vi "ActionVIOnCompile.vi"(8 "error in (no error)":errorcluster, 11 "Device Item Ref in":T1 format="%.0x") -> (0 "error out":errorcluster)   [LabVIEW 2011, in "Chassis TimeSync System Explorer.lvlib"]
uses:
  Chassis TimeSync System Explorer.lvlib
  <vilib>/NI Veristand/Custom Device API/Custom Device Item Ref.ctl
  Shared/Compiled Data.ctl
  Shared/Connection Settings.ctl
  Shared/Mode.ctl
  Shared/External Pin.ctl
  Shared/Routes.ctl
  Shared/Route.ctl
  Shared/Time Ref Settings.ctl
  Shared/Time Reference.ctl
  Shared/IRIG Type.ctl
  Shared/Constants.vi
  <vilib>/NI Veristand/Custom Device API/Get Item Property (String).vi
  <vilib>/NI Veristand/Custom Device API/Get Item Property (U16).vi
  <vilib>/NI Veristand/Custom Device API/Get Item Property (Double).vi
  <vilib>/NI Veristand/Custom Device API/Get Item Property (Boolean).vi
  <vilib>/NI Veristand/Custom Device API/Set Item Property (Variant).vi
  Shared/Chassis TimeSync Shared.lvlib
  <vilib>/NI Veristand/Custom Device API/Custom Device API.lvlib
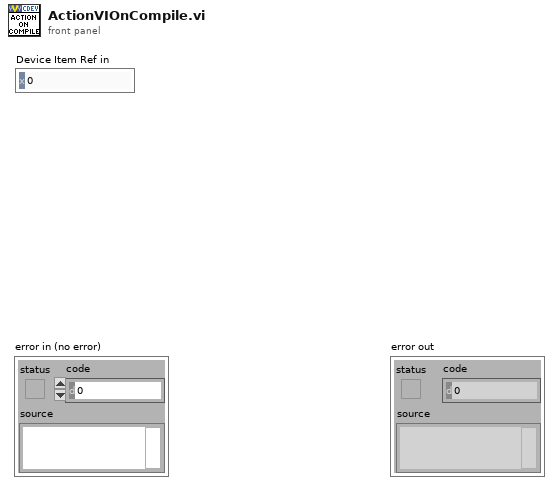
[diagram p1: front panel]
types:
  T1 = typedef "Custom Device API.lvlib/Custom Device Item Ref.ctl" = u64
  T2 = typedef "Chassis TimeSync Shared.lvlib/Compiled Data.ctl" = cluster{"SyncMod?":bool, "SyncMod":string, "ConnectionSettings":T3, "TimeKeeper":string, "ScanOffset(%)":dbl, "StartDelay(s)":u16, "Time Ref Settings":T8, "FIFO Locations":cluster{"SysTime":i32[], "TimeRef":i32[], "Status":i32[]}}
  T3 = typedef "Chassis TimeSync Shared.lvlib/Connection Settings.ctl" = cluster{"Mode":T4, "pxitrig":bool, "pfi0":bool, "pfi1":bool, "pfi2":bool, "External Pin":T5, "Routes":T6}
  T4 = typedef "Chassis TimeSync Shared.lvlib/Mode.ctl" = enum16{"Generate sample clock", "Route sample clock out of chassis", "Route sample clock into chassis", "Custom routes"}
  T5 = typedef "Chassis TimeSync Shared.lvlib/External Pin.ctl" = enum16{"PFI0", "PFI1", "PFI2"}
  T6 = typedef "Chassis TimeSync Shared.lvlib/Routes.ctl" = T7[]
  T7 = typedef "Chassis TimeSync Shared.lvlib/Route.ctl" = cluster{"Source":string, "Destination":string}
  T8 = typedef "Chassis TimeSync Shared.lvlib/Time Ref Settings.ctl" = cluster{"Time Reference":T9, "Priority 1":i32, "Priority 2":i32, "IRIG type":T10, "Terminal":string, "PPSSetTime":bool, "Start Time":timestamp}
  T9 = typedef "Chassis TimeSync Shared.lvlib/Time Reference.ctl" = enum16{"GPS", "IRIG", "PPS", "1588 Ordinary Clock", "PXI Chassis Clock"}
  T10 = typedef "Chassis TimeSync Shared.lvlib/IRIG Type.ctl" = enum16{"IRIGB DC", "IRIGB AM"}
  T11 = typedef "Chassis TimeSync Shared.lvlib/Channel.ctl" = cluster{"Name":string, "Units":string, "Default":dbl, "Description":string}
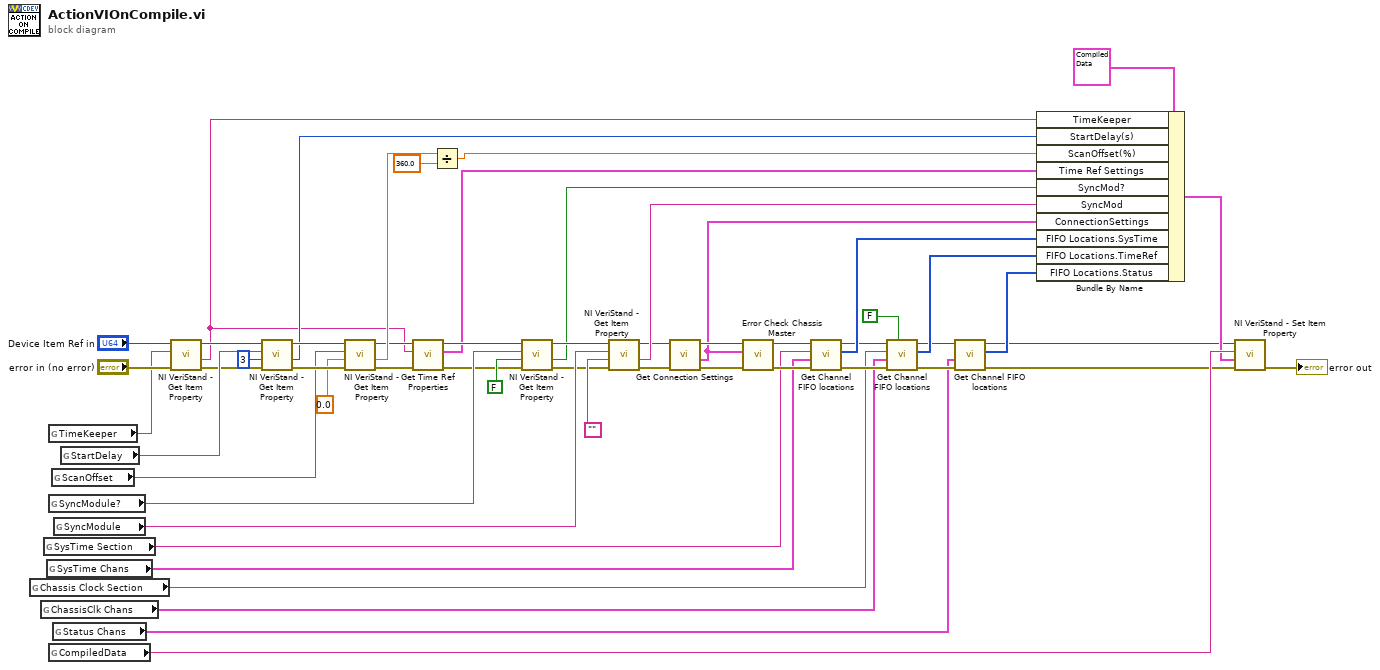
[diagram p0: block diagram]
diagram:
  n1 = global read "Constants.vi" "Chassis Clock Section"() -> (w11:string)
  n2 = global read "Constants.vi" "ChassisClk Chans"() -> (w10:T11[])
  n3 = global read "Constants.vi" "SysTime Section"() -> (w15:string)
  n4 = global read "Constants.vi" "SysTime Chans"() -> (w16:T11[])
  n5 = global read "Constants.vi" "TimeKeeper"() -> (w53:string)
  n6 = global read "Constants.vi" "SyncModule?"() -> (w37:string)
  n7 = global read "Constants.vi" "CompiledData"() -> (w20:string)
  n8 = global read "Constants.vi" "ScanOffset"() -> (w48:string)
  n9 = global read "Constants.vi" "Status Chans"() -> (w6:T11[])
  n10 = global read "Constants.vi" "SyncModule"() -> (w35:string)
  n11 = global read "Constants.vi" "StartDelay"() -> (w50:string)
  n12 = call-poly <vilib>:"NI VeriStand - Get Item Property.vi"("error in (no error)"="error in (no error)", "Property Name"=w53, "Item Ref in"="Device Item Ref in") -> ("error out"=w46:errorcluster, "Value"=w38:string, "Item Ref out"=w45:T1)  [unwired: 5 in, 1 out]
  n13 = call-poly <vilib>:"NI VeriStand - Get Item Property.vi"("error in (no error)"=w46, "Default Value"=u16 3 ("Start Offset Multiple"), "Property Name"=w50, "Item Ref in"=w45) -> ("error out"=w51:errorcluster, "Value"=w44:u16, "Item Ref out"=w52:T1)  [unwired: 4 in, 1 out]
  n14 = call-poly <vilib>:"NI VeriStand - Get Item Property.vi"("error in (no error)"=w51, "Default Value"=0.0 ("Scan Offset Scale (%)"), "Property Name"=w48, "Item Ref in"=w52) -> ("error out"=w40:errorcluster, "Value"=w43:dbl, "Item Ref out"=w39:T1)  [unwired: 4 in, 1 out]
  n15 = call "Get Time Ref Properties.vi"("error in (no error)"=w40, "TimeKeeper Module"=w38, "Device Item Ref in"=w39) -> ("error out"=w33:errorcluster, "Time Ref Settings"=w26:T8, "Item Ref out"=w32:T1)  [unwired: 6 in]
  n16 = Divide(x=w43, y=360.0) -> (x/y=w42:dbl)
  n17 = call-poly <vilib>:"NI VeriStand - Get Item Property.vi"("error in (no error)"=w33, "Default Value"=FALSE, "Property Name"=w37, "Item Ref in"=w32) -> ("error out"=w30:errorcluster, "Value"=w29:bool, "Item Ref out"=w31:T1)  [unwired: 4 in, 1 out]
  n18 = call-poly <vilib>:"NI VeriStand - Get Item Property.vi"("error in (no error)"=w30, "Default Value"="", "Property Name"=w35, "Item Ref in"=w31) -> ("error out"=w27:errorcluster, "Value"=w28:string, "Item Ref out"=w24:T1)  [unwired: 4 in, 1 out]
  n19 = call "Get Connection Settings.vi"("error in (no error)"=w27, "Item Ref in"=w24) -> ("error out"=w25:errorcluster, "Connection Settings"=w22:T3, "Item Ref out"=w23:T1)  [unwired: 6 in, 1 out]
  n20 = call "Error Check Chassis Master.vi"("error in (no error)"=w25, "Connection Settings"=w22, "Item Ref in"=w23) -> ("error out"=w18:errorcluster, "Item Ref out"=w17:T1)  [unwired: 7 in]
  n21 = call "Get Channel FIFO locations.vi"("error in (no error)"=w18, "Channels to get refs"=w16, "Section By Relative Path (\"\")"=w15, "Device Ref in"=w17) -> ("error out"=w13:errorcluster, "FIFO Locations"=w14:i32[], "Device Ref out"=w12:T1)  [unwired: 5 in]
  n22 = call "Get Channel FIFO locations.vi"("Error On Missing Section? (T)"=FALSE, "error in (no error)"=w13, "Channels to get refs"=w10, "Section By Relative Path (\"\")"=w11, "Device Ref in"=w12) -> ("error out"=w8:errorcluster, "FIFO Locations"=w9:i32[], "Device Ref out"=w7:T1)  [unwired: 4 in]
  n23 = call "Get Channel FIFO locations.vi"("error in (no error)"=w8, "Channels to get refs"=w6, "Device Ref in"=w7) -> ("error out"=w4:errorcluster, "FIFO Locations"=w5:i32[], "Device Ref out"=w3:T1)  [unwired: 6 in]
  n24 = Bundle By Name(cluster=T2 {"SyncMod?"=FALSE, "SyncMod"="", "ConnectionSettings"={"Mode"=enum."Generate sample clock", "pxitrig"=FALSE, "pfi0"=FALSE, "pfi1"=FALSE, "pfi2"=FALSE, "External Pin"=enum."PFI0", "Routes"=[]}, "TimeKeeper"="", "ScanOffset(%)"=0.0, "StartDelay(s)"=0, "Time Ref Settings"={"Time Reference"=enum."GPS", "Priority 1"=0, "Priority 2"=0, "IRIG type"=enum."IRIGB AM", "Terminal"="", "PPSSetTime"=FALSE, "Start Time"=timestamp(0 s since 1904-01-01)}, "FIFO Locations"={"SysTime"=[], "TimeRef"=[], "Status"=[]}} ("Compiled Data"), "TimeKeeper"=w38, "StartDelay(s)"=w44, "ScanOffset(%)"=w42, "Time Ref Settings"=w26, "SyncMod?"=w29, "SyncMod"=w28, "ConnectionSettings"=w22, "FIFO Locations.SysTime"=w14, "FIFO Locations.TimeRef"=w9, "FIFO Locations.Status"=w5) -> (w19:T2)
  n25 = call-poly <vilib>:"NI VeriStand - Set Item Property.vi"("error in (no error)"=w4, "Value"=w19, "Property Name"=w20, "Item Ref in"=w3) -> ("error out"=→"error out":errorcluster)  [unwired: 5 in, 2 out]
